vi "Calculate Stt.vi"(11 "N":i64) -> (2 "St":i64, 3 "Stt":i64)   [LabVIEW 2015]
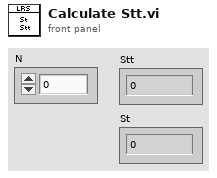
[diagram p1: front panel]
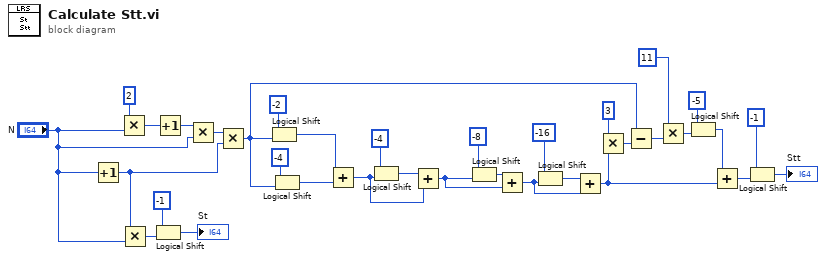
[diagram p0: block diagram]
diagram:
  n1 = Increment(x="N") -> (x+1=w3:i64)
  n2 = Multiply(x=i64 2 ("y"), y="N") -> (x*y=w31:i64)
  n3 = Multiply(x=w3, y="N") -> (x*y=w5:i64)
  n4 = Logical Shift(y=i16 -1, x=w5) -> (x << y=→"St":i64)
  n5 = Increment(x=w31) -> (x+1=w32:i64)
  n6 = Multiply(x=w32, y="N") -> (x*y=w33:i64)
  n7 = Multiply(x=w33, y=w3) -> (x*y=w21:i64)
  n8 = Logical Shift(y=i16 -2, x=w21) -> (x << y=w8:i64)
  n9 = Logical Shift(y=i16 -4, x=w21) -> (x << y=w9:i64)
  n10 = Add(x=w8, y=w9) -> (x+y=w12:i64)
  n11 = Logical Shift(y=i16 -4, x=w12) -> (x << y=w11:i64)
  n12 = Add(x=w11, y=w12) -> (x+y=w15:i64)
  n13 = Logical Shift(y=i16 -8, x=w15) -> (x << y=w14:i64)
  n14 = Add(x=w14, y=w15) -> (x+y=w18:i64)
  n15 = Logical Shift(y=i16 -16, x=w18) -> (x << y=w17:i64)
  n16 = Add(x=w17, y=w18) -> (x+y=w27:i64)
  n17 = Multiply(x=i64 3 ("y"), y=w27) -> (x*y=w20:i64)
  n18 = Subtract(x=w21, y=w20) -> (x-y=w24:i64)
  n19 = Multiply(x=i64 11 ("y"), y=w24) -> (x*y=w25:i64)
  n20 = Logical Shift(y=i16 -5, x=w25) -> (x << y=w26:i64)
  n21 = Add(x=w26, y=w27) -> (x+y=w28:i64)
  n22 = Logical Shift(y=i16 -1, x=w28) -> (x << y=→"Stt":i64)
